vi "Init DO DAQ.vi"(0 "DaqDevice":string="USB6212", 7 "DO LineList":string[](array[string])=["port1/line4:7", "port2/line0:7"], 11 "error in":errorcluster, 12 "instance":i32) -> (8 "DO task":refnum<k21>, 15 "error out":errorcluster)   [LabVIEW 2017]
doc: "Developed by Kevin Thompson\nThompson Engineering, LLC\nkevin@thompsonengineering.net"
uses:
  <vilib>/DAQmx/create/channels.llb/DAQmx Create Channel (DO-Digital Output).vi
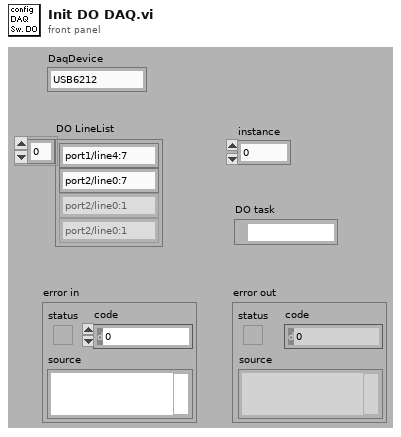
[diagram p1: front panel]
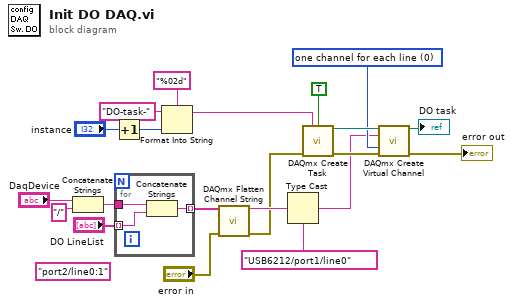
[diagram p0: block diagram]
diagram:
  (unwired) "port2/line0:1"
  w17 = 0 items=["one channel for each line", "one channel for all lines"] ("line grouping")
  n1 = Concatenate Strings("DaqDevice", "/") -> (w11:string)
  n2 = Increment(x="instance") -> (x+1=w2:i32)
  n3 = for {
    tunnel: "DO LineList" -> [w23] mode=indexing
    tunnel: w11 -> [w24]
    tunnel: [w22] -> w10 mode=indexing
    n4 = Concatenate Strings(w24, w23) -> (w22:string)
  }
  n5 = Format Into String(format string="%02d", initial string="DO-task-", w2) -> (resulting string=w1:string)  [unwired: 1 in, 1 out]
  n6 = call <vilib>:"DAQmx Flatten Channel String.vi"("names in"=w10, "error in"="error in") -> ("names out"=w8:string, "error out"=w7:errorcluster)  [unwired: 12 in]
  n7 = Type Cast(type=tag "USB6212/port1/line0" ("lines"), x=w8) -> (*(type *) &x=w16:tag)
  n8 = call <vilib>:"DAQmx Create Task.vi"("new task name"=w1, "auto cleanup"=TRUE, "error in"=w7) -> ("task out"=w19:refnum<k21>, "error out"=w20:errorcluster)  [unwired: 11 in]
  n9 = call-poly <vilib>:"DAQmx Create Virtual Channel.vi"("task in"=w19, "lines"=w16, "line grouping"=w17, "error in"=w20) -> ("task out"=→"DO task":refnum<k21>, "error out"=→"error out":errorcluster)  [unwired: 10 in]
